vi "writeRPDO.vi"(7 "RPDO data":u8[](array[numeric])=[0, 0, 0, 0, 0, 0, 0, 0], 8 "error in (no error)":errorcluster, 9 "PDOChannel":u8(ring) items=["PDO 1", "PDO 2", "PDO 3", "PDO 4"], 10 "interface object in":refnum<k20>, 11 "MotorControllerClass in":refnum<class "MotorControllerClass.lvclass">) -> (0 "error out":errorcluster, 2 "interface object out":refnum<k20>, 3 "MotorControllerClass out":refnum<class "MotorControllerClass.lvclass">)   [LabVIEW 2018, in "MotorControllerClass.lvclass"]
uses:
  BMS/MotorControllerClass.lvclass
  <vilib>/CANopenLib/CANOPEN.llb/CANopen RPDO Create.vi
  <vilib>/CANopenLib/CANOPEN.llb/CANopen RPDO Start.vi
  <vilib>/CANopenLib/CANOPEN.llb/CANopen RPDO Close.vi
  <resource>/objmgr/CANopenPDO.rc
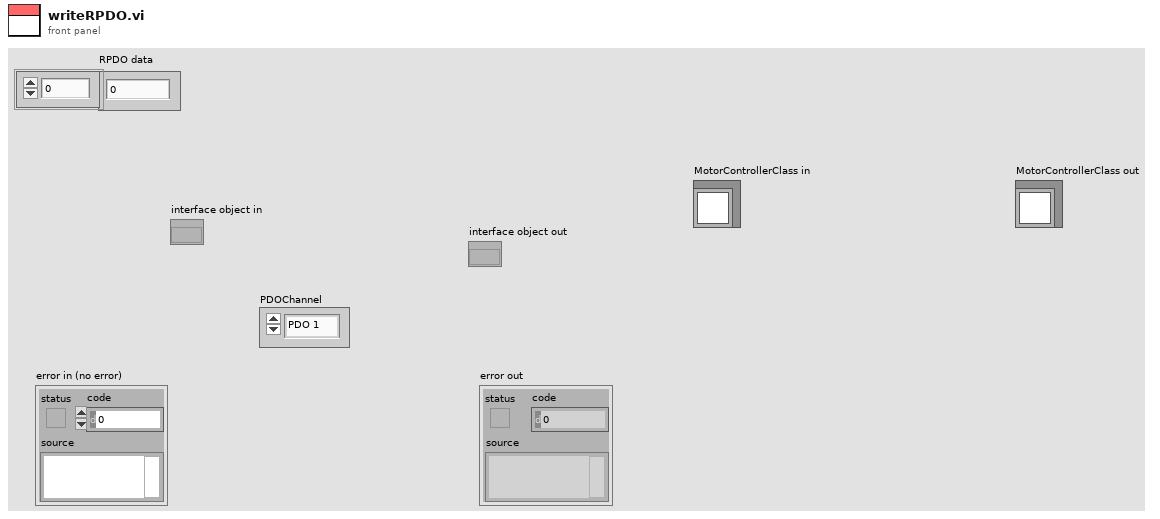
[diagram p1: front panel]
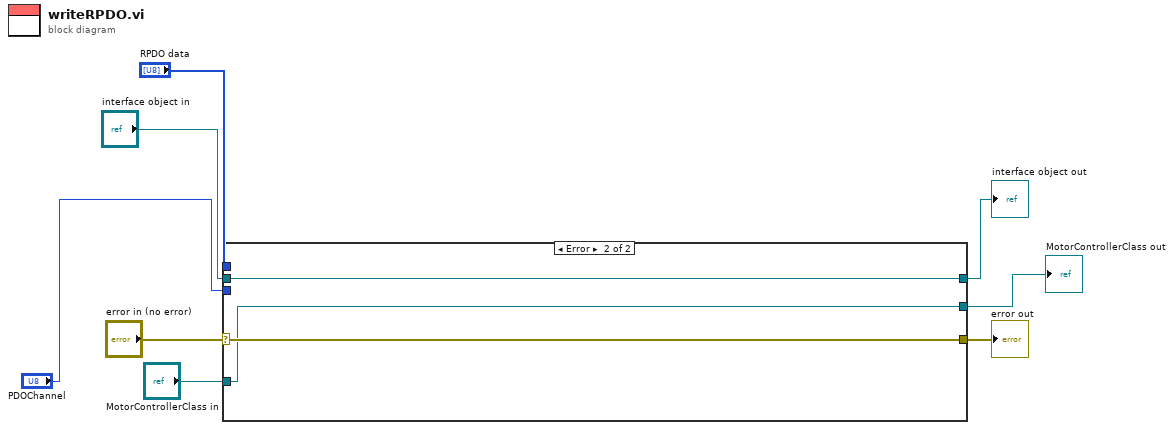
[diagram p0: block diagram]
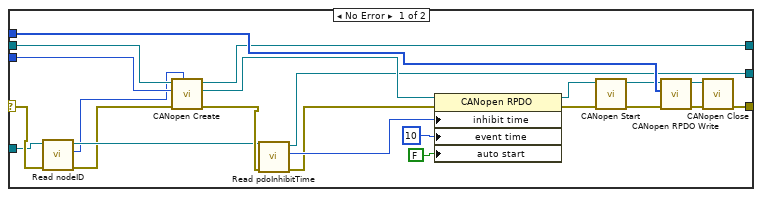
[diagram p2: hidden frame]
diagram:
  n1 = case shown="Error" "error in (no error)" {
    selector: "error in (no error)" -> [w11 w34]
    tunnel: [w21 w34] -> w7
    tunnel: [w18 w33] -> w6
    tunnel: "interface object in" -> [w31 w33]
    tunnel: "PDOChannel" -> [w30 _]
    tunnel: "RPDO data" -> [w23 _]
    tunnel: "MotorControllerClass in" -> [w10 w32]
    tunnel: [w9 w32] -> w1
    frame No Error {
      n2 = call-dynamic "Read nodeID.vi"("error in (no error)"=w11, "MotorControllerClass in"=w10) -> ("error out"=w12:errorcluster, "nodeID"=w13:u8, "MotorControllerClass out"=w14:refnum<class "MotorControllerClass.lvclass">)  [unwired: 7 in]
      n3 = call-poly <vilib>:"CANopen Create.vi"("node-ID"=w13, "error in (no error)"=w12, "PDO channel"=w30, "interface object in"=w31) -> ("error out"=w15:errorcluster, "RPDO object out"=w29:refnum<k20>, "interface object out"=w18:refnum<k20>)  [unwired: 5 in]
      n4 = call-dynamic "Read pdoInhibitTime.vi"("error in (no error)"=w15, "MotorControllerClass in"=w14) -> ("error out"=w16:errorcluster, "pdoInhibitTime"=w17:u8, "MotorControllerClass out"=w9:refnum<class "MotorControllerClass.lvclass">)  [unwired: 7 in]
      n5 = property class="CANopen RPDO"(reference=w29, error in=w16, "inhibit time"=w17, "event time"=u8 10, "auto start"=FALSE) -> (reference out=w25:refnum<k20>, error out=w26:errorcluster)
      n6 = call-poly <vilib>:"CANopen Start.vi"("error in (no error)"=w26, "RPDO object in"=w25) -> ("error out"=w24:errorcluster, "RPDO object out"=w22:refnum<k20>)  [unwired: 8 in]
      n7 = call <vilib>:"CANopen RPDO Write.vi"("error in (no error)"=w24, "data"=w23, "RPDO object in"=w22) -> ("error out"=w20:errorcluster, "RPDO object out"=w19:refnum<k20>)  [unwired: 7 in]
      n8 = call-poly <vilib>:"CANopen Close.vi"("error in (no error)"=w20, "RPDO object in"=w19) -> ("error out"=w21:errorcluster)  [unwired: 9 in]
    }
    frame Error {
    }
  }
  "error out" <- w7
  "interface object out" <- w6
  "MotorControllerClass out" <- w1
